vi "CollectDataAndSave.vi"(0 "SPC DLL Path":path, 1 "CycleNo":i32, 2 "Storing Path":path, 5 "Module No":i16, 11 "error in":errorcluster, 12 "SPC memory config":T1 {"Frames Per Page" min=1 step=1; "Maxpage" min=1; "Blocks Per Frame" min=1 step=1}, 13 "#Curves":i32, 14 "Serialnumber\nper Module":string) -> (3 "stored to":string, 4 "SPC DLL Path":path, 6 "Module No":i16, 10 "Data":u16[][](array[numeric]), 15 "error out":errorcluster)   [LabVIEW 2017]
doc: "This convenience VIs wraps SPC_read_data_page.vi and SPC_save_data_to_sdtfile.vi in one VI to provide a clearer code.\n\n<b>Note:</b> This VI is set to execute as preallocated clone to improve performance when run in parallel loops for multi module setups.\n\ninfo@becker-hickl.com"
uses:
  SPC_Wrappers/SPC_Controls/ConfigMem.ctl
panel:
  out "DataGraph":cluster{"Waveform Graph":u16[]}[](array[cluster])
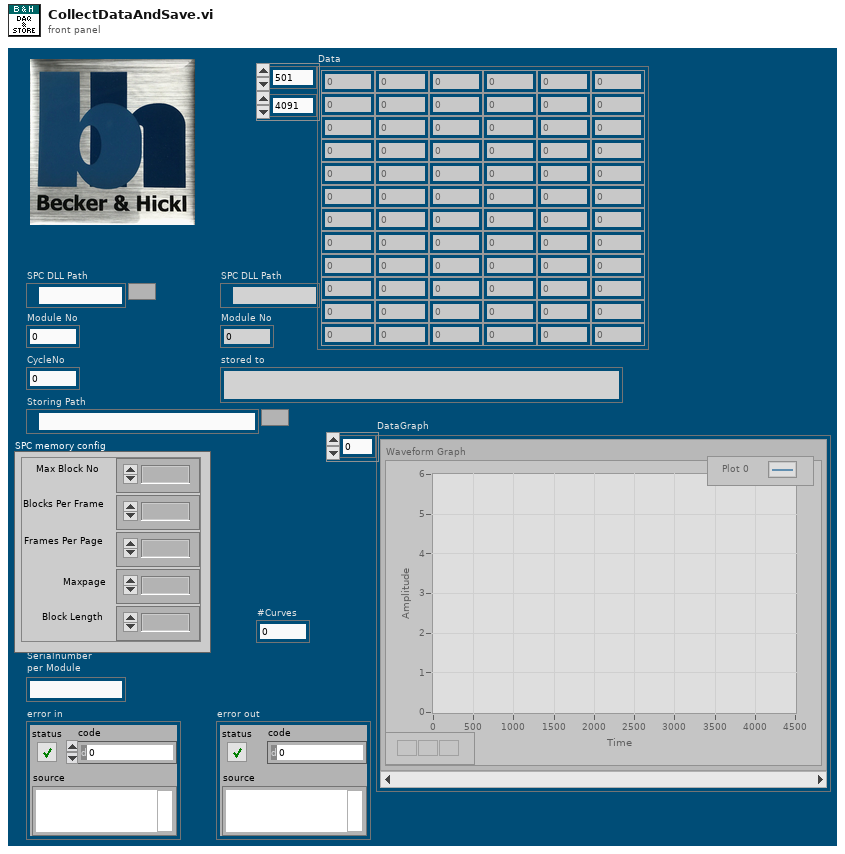
[diagram p1: front panel]
types:
  T1 = typedef "ConfigMem.ctl" = cluster{"Max Block No":i32, "Blocks Per Frame":i32, "Frames Per Page":i32, "Maxpage":i32, "Block Length":i32}
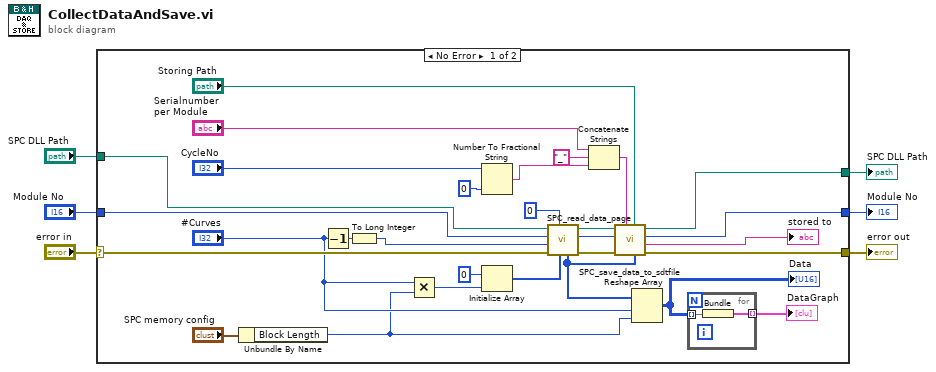
[diagram p0: block diagram]
diagram:
  n1 = case shown="No Error" "error in" {
    selector: "error in" -> [w17 w40]
    tunnel: [w35 w40] -> w6
    tunnel: "SPC DLL Path" -> [w21 w39]
    tunnel: "Module No" -> [w20 w38]
    tunnel: [w19 w39] -> w2
    tunnel: [w18 w38] -> w1
    frame No Error {
      n2 = Unbundle By Name("SPC memory config") -> ("Block Length"=w7:i32)
      n3 = Decrement(x="#Curves") -> (x-1=w27:i32)
      n4 = To Long Integer(number=w27) -> (32bit integer=w29:i32)
      n5 = Multiply(x="#Curves", y=w7) -> (x*y=w28:i32)
      n6 = Number To Fractional String(number="CycleNo", precision (6)=i16 0) -> (F-format string=w34:string)  [unwired: 2 in]
      n7 = Initialize Array(u16 0, w28) -> (w11:u16[])
      n8 = call "SPC_read_data_page.vi"("DataBuffer"=w11, "First Page"=0, "Error In"=w17, "Last Page"=w29, "Module No"=w20, "DLL Path"=w21) -> ("Error Out"=w30:errorcluster, "Module No"=w25:i16, "DLL Path"=w24:path, "Output Data"=w12:u16[])  [unwired: 2 in]
      n9 = Concatenate Strings("Serialnumber\nper Module", "_", w34) -> (w13:string)
      n10 = call "SPC_save_data_to_sdtfile.vi"("Data"=w12, "Storing Path"="Storing Path", "SDT File Name"=w13, "Error In"=w30, "Module No"=w25, "DLL Path"=w24) -> ("Error Out"=w35:errorcluster, "Stored to"=→"stored to":string, "Module No"=w18:i16, "DLL Path"=w19:path)  [unwired: 2 in]
      n11 = Reshape Array(w12, "#Curves", w7) -> (w9:u16[][])
      "Data" <- w9
      n12 = for {
        tunnel: w9 -> [w36] mode=indexing
        tunnel: [w37] -> w8 mode=indexing
        n13 = Bundle("Output Data"=w36) -> (w37:cluster{"Output Data":u16[]})  [unwired: 1 in]
      }
      "DataGraph" <- w8
    }
    frame Error {
    }
  }
  "error out" <- w6
  "Module No" <- w1
  "SPC DLL Path" <- w2
